vi "Actor Core.vi"(8 "error in":errorcluster, 11 "UDP Reader in":refnum<class "UDP Reader.lvclass">) -> (0 "error out":errorcluster, 3 "Actor out":refnum<class "Actor.lvclass">)   [LabVIEW 2022 SP3, in "UDP Reader.lvlib" / "UDP Reader.lvclass"]
doc: "(<B>Filename</B>: Actor Framework.lvlib:Actor.lvclass:Actor Core.vi)\n\nReceives messages to the actor, reacts to them, and initiates any error handling that may shut the actor down.\n\nDescendant classes may override this VI to append parallel tasks for the actor to complete while it handles messages. Overrides use the Call Parent Class Method node."
uses:
  UDP Reader.lvclass
  C:/Program Files (x86)/National Instruments/LabVIEW 2022/vi.lib/ActorFramework/Actor/Actor.lvclass
  <vilib>/ActorFramework/Actor/Actor.lvclass
  UDP Input.ctl
  UDP Reader Messages/Read Msg/Read Msg.lvclass
  C:/Program Files (x86)/National Instruments/LabVIEW 2022/vi.lib/ActorFramework/Message/Message.lvclass
  UDP Reader Messages/Feedback Msg/Feedback Msg.lvclass
  <vilib>/ActorFramework/Message Enqueuer/Message Priority.ctl
  UDP Reader.lvclass/UDP Reader.ctl
  <vilib>/ActorFramework/Actor/Actor.lvclass/Actor.ctl
  <vilib>/ActorFramework/Message Enqueuer/Message Enqueuer.lvclass/Message Enqueuer.ctl
  <vilib>/ActorFramework/Message Enqueuer/Init from Existing Queue.vi
  <vilib>/ActorFramework/Message Enqueuer/Enqueue.vi
  UDP Reader Messages/Reconnect Msg/Reconnect Msg.lvclass
  <vilib>/ActorFramework/Stop Msg/Stop Msg.lvclass
  <vilib>/ActorFramework/Message Priority Queue/Priority Enqueue.vi
  <vilib>/MGI/Monitored Actor/Monitored Actor/Monitored Actor/Monitored Actor.lvclass
  <vilib>/ActorFramework/Message Enqueuer/Message Enqueuer.lvclass
  C:/Users/ebert/Documents/codes/ssl/repo/teste/UDP Reader/UDP Reader Messages/Feedback Msg/Feedback Msg.lvclass
  C:/Program Files (x86)/National Instruments/LabVIEW 2022/vi.lib/MGI/Monitored Actor/Monitored Actor/Monitored Actor/Monitored Actor.lvclass
  C:/Users/ebert/Documents/codes/ssl/repo/teste/UDP Reader/UDP Reader/UDP Reader.lvclass
  C:/Users/ebert/Documents/codes/ssl/repo/teste/UDP Reader/UDP Reader Messages/Read Msg/Read Msg.lvclass
panel:
  in  "stop":bool
  out "Connection ID":refnum<k16>
  out "Input":T1
  out "Data":u8[](array[numeric])
  out "Error":bool
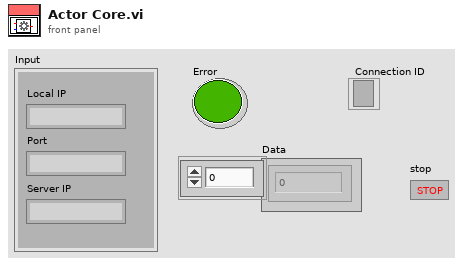
[diagram p1: front panel]
types:
  T1 = typedef "UDP Input.ctl" = cluster{"Local IP":string, "Port":string, "Server IP":string}
  T2 = typedef "Actor Framework.lvlib/Message Enqueuer.lvclass/Message Priority.ctl" = enum16{"Low", "Normal", "High"}
  T3 = cluster{"Stop":refnum<user-event>, "Reconnect":refnum<user-event>}
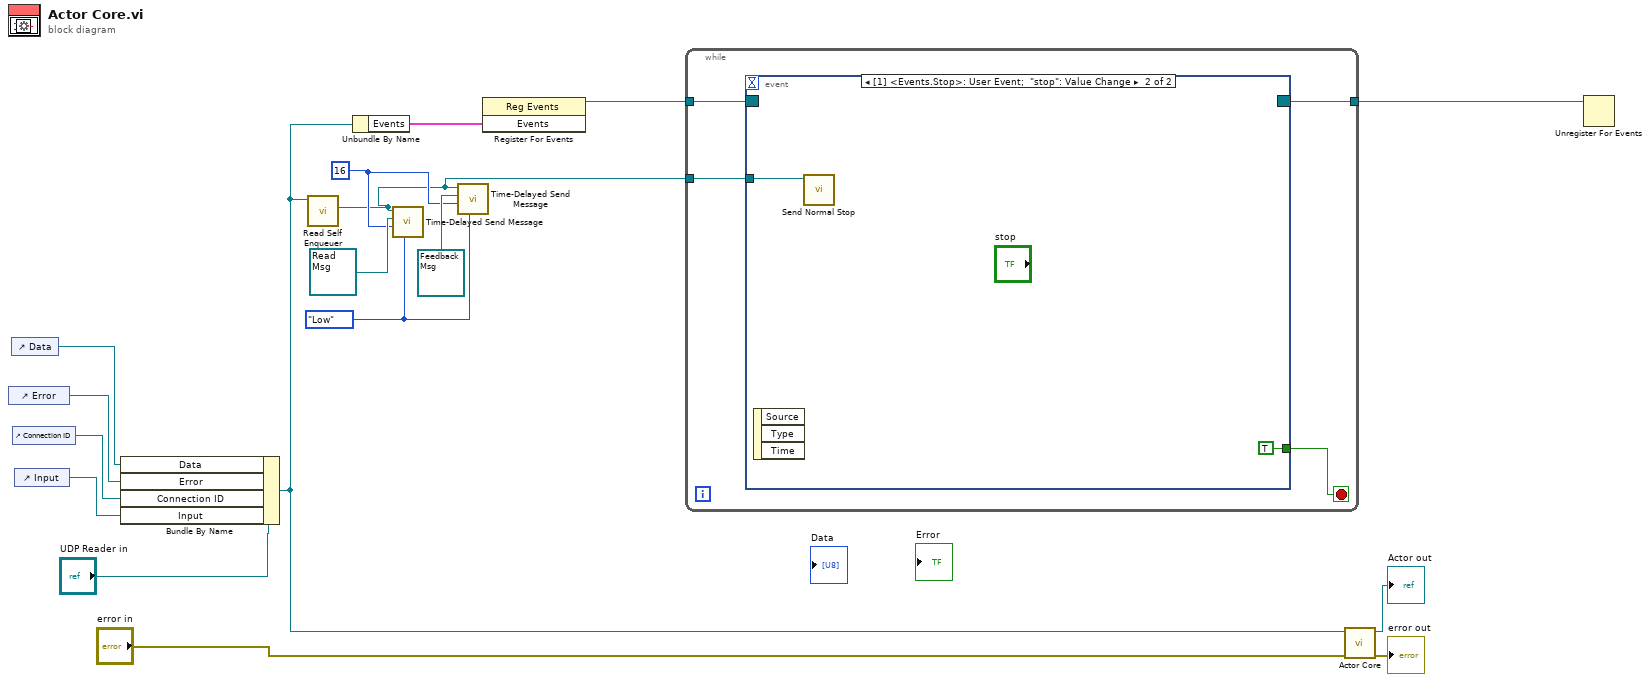
[diagram p0: block diagram]
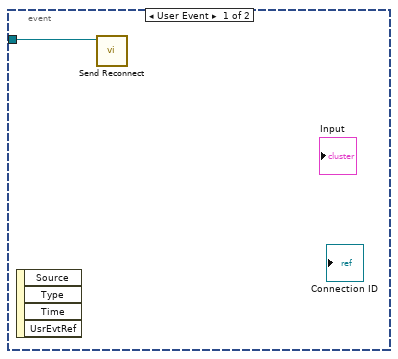
[diagram p2: hidden frame]
diagram:
  w2 = Message_Priority."Low" ("Message Priority (Normal)")
  w3 = 16 ("Milliseconds To Wait")
  n1 = control-ref of="Error"() -> (w8:refnum<vi>)
  n2 = control-ref of="Data"() -> (w9:refnum<vi>)
  n3 = control-ref of="Connection ID"() -> (w7:refnum<vi>)
  n4 = control-ref of="Input"() -> (w6:refnum<vi>)
  n5 = Bundle By Name(cluster="UDP Reader in", "Data"=w9, "Error"=w8, "Connection ID"=w7, "Input"=w6) -> (w10:refnum<class "UDP Reader.lvclass">)
  n6 = call <vilib>:"Read Self Enqueuer.vi"("Actor"=w10) -> ("Self Enqueuer"=w1:refnum<class "Message Enqueuer.lvclass">)  [unwired: 10 in]
  n7 = Unbundle By Name(w10) -> ("Events"=w13:T3)
  n8 = call <vilib>:"Time-Delayed Send Message.vi"("Message Priority (Normal)"=w2, "Milliseconds To Wait"=w3, "Message"=refnum<class "Read Msg.lvclass"> refnum ("UDP Reader.lvlib:Read Msg.lvclass"), "Message Enqueuer"=w1) -> ()  [unwired: 6 in, 2 out]
  n9 = call <vilib>:"Time-Delayed Send Message.vi"("Message Priority (Normal)"=w2, "Milliseconds To Wait"=w3, "Message"=refnum<class "Feedback Msg.lvclass"> refnum ("UDP Reader.lvlib:Feedback Msg.lvclass"), "Message Enqueuer"=w1) -> ()  [unwired: 6 in, 2 out]
  n10 = register-events(w13) -> (reference out=w14:refnum<event-registration>)  [unwired: 2 in, 1 out]
  n11 = while {
    tunnel: w14 -> [w21]
    tunnel: [w20] -> w12
    tunnel: w1 -> [w18]
    stop <- w19 stop-if-true
    n12 = event shown="[1] <Events.Stop>: User Event;  \"stop\": Value Change" {
      selector: w21 -> [_ _]
      dyn-events: [_ _] -> w20
      timeout: _ -> [_ _]
      tunnel: [_ TRUE] -> w19
      tunnel: w18 -> [w22 w23]
      event User Event {
        n13 = event-data() -> ()  [unwired: 1 in, 4 out]
        n14 = call "Send Reconnect.vi"("Message Enqueuer in"=w22) -> ()  [unwired: 9 in, 2 out]
      }
      event User Event; "stop": Value Change {
        n15 = event-data() -> ()  [unwired: 1 in, 3 out]
        n16 = call <vilib>:"Send Normal Stop.vi"("Message Enqueuer"=w23) -> ()  [unwired: 10 in, 1 out]
      }
    }
  }
  n17 = call-parent "Actor Core.vi"("error in"="error in", "Actor in"=w10) -> ("error out"=→"error out":errorcluster, "Actor out"=→"Actor out":refnum<class "Actor.lvclass">)  [unwired: 8 in]
  n18 = Unregister For Events(event registration refnum=w12) -> ()  [unwired: 1 in, 1 out]
